vi "Save script file.vi"(10 "Multiplication factor":u16, 11 "Script Array":T1[](array[typedef]) {"Carousel" items=["0", "1", "2", "3", "4", "5", "6"]; "Angle [°]" min=0.0 max=350.0; "Tau [ms]" min=0.0 max=100.0; "Wait [min]" min=0.0 max=3000.0; "Tmp [K]" min=0.0 max=3000.0; "Mod_A [G]" min=0.1 max=150.0; "Mod_F [kHz]" min=0.1 max=150.0}) -> ()   [LabVIEW 2024]
uses:
  Datatypes/script polymorh line.ctl
  <vilib>/Utility/config.llb/Write Key (I32).vi
  <vilib>/Utility/config.llb/Write Key (U32).vi
  <vilib>/Utility/config.llb/NI_LVConfig.lvlib
  <userlib>/_OpenG.lib/variantconfig/variantconfig.llb/openg_variant_configuration_file.lvlib
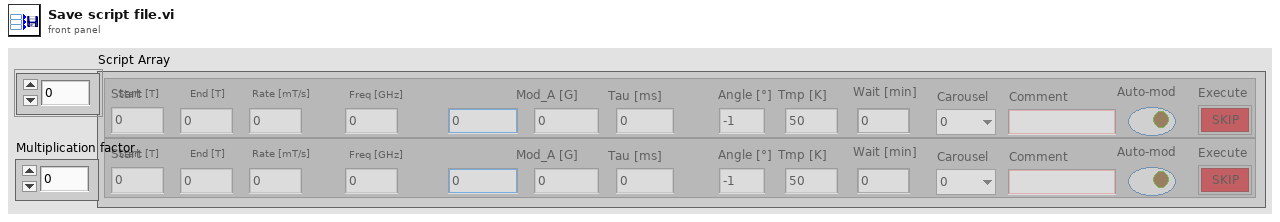
[diagram p1: front panel]
types:
  T1 = typedef "script polymorh line.ctl" = cluster{"Start":dbl, "Start Caption":string, "End":dbl, "End Caption":string, "Sweep":dbl, "Sweep caption":string, "Constant":dbl, "Constant caption":string, "Mod_F [kHz]":dbl, "Mod_A [G]":dbl, "Tau [ms]":dbl, "Angle [°]":dbl, "Tmp [K]":dbl, "Wait [min]":dbl, "Carousel":i8, "Comment":string, "Auto-mod":bool, "Execute":bool}
  T2 = typedef "NI_LVConfig.lvlib/Config Data RefNum.ctl" = refnum<k1>
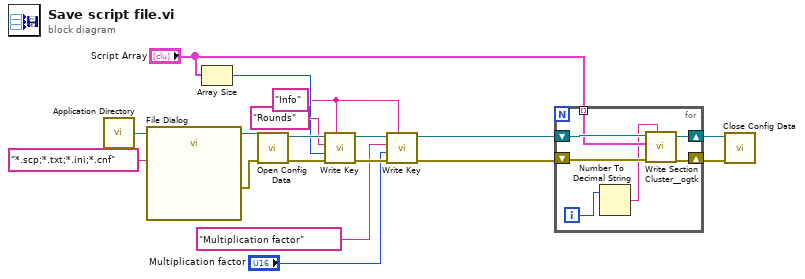
[diagram p0: block diagram]
diagram:
  w3 = "Info" ("section")
  n1 = call <vilib>:"Application Directory.vi"() -> ("Application Directory"=w15:path)
  n2 = call "File Dialog"("start path"=w15, "pattern (all files)"="*.scp;*.txt;*.ini;*.cnf" ("string")) -> ("selected path"=w14:path, "error out"=w16:errorcluster)  [unwired: 10 in, 2 out]
  n3 = Array Size(array="Script Array") -> (size(s)=w9:i32)
  n4 = call <vilib>:"Open Config Data.vi"("error in (no error)"=w16, "configuration file path"=w14) -> ("error out"=w8:errorcluster, "refnum"=w12:T2)  [unwired: 7 in, 1 out]
  n5 = call-poly <vilib>:"Write Key.vi"("section"=w3, "error in (no error)"=w8, "value"=w9, "key"="Rounds", "refnum"=w12) -> ("error out"=w5:errorcluster, "refnum out"=w7:T2)  [unwired: 4 in, 1 out]
  n6 = call-poly <vilib>:"Write Key.vi"("section"=w3, "error in (no error)"=w5, "value"="Multiplication factor", "key"="Multiplication factor", "refnum"=w7) -> ("error out"=w4:errorcluster, "refnum out"=w6:T2)  [unwired: 4 in, 1 out]
  n7 = for {
    tunnel: "Script Array" -> [w21] mode=indexing
    shift-right: [w25] -> w18
    shift-left: w4 -> [w23]
    shift-right: [w24] -> w17
    shift-left: w6 -> [w22]
    i -> [w20]
    n8 = Number To Decimal String(number=w20) -> (decimal integer string=w19:string)  [unwired: 1 in]
    n9 = call <userlib>:"Write Section Cluster__ogtk.vi"("section (optional)"=w19, "error in (no error)"=w23, "Section Formatted Cluster"=w21, "refnum"=w22) -> ("error out"=w25:errorcluster, "dup refnum"=w24:T2)  [unwired: 6 in]
  }
  n10 = call <vilib>:"Close Config Data.vi"("error in (no error)"=w18, "refnum"=w17) -> ()  [unwired: 8 in, 2 out]
